vi "PusherClose.vi"   [LabVIEW 2014, in "PusherLib.lvlib"]
uses:
  PusherLib.lvlib
  PusherRefs.ctl
types:
  T1 = typedef "PusherLib.lvlib/PusherRefs.ctl" = enum16{"PusherLeft", "PusherRight", "PusherStringPot"}
  T2 = typedef "WPI_MotorControlDeviceRef.ctl" = cluster{"DeviceStatus":errorcluster, "Type":T3, "PWM":cluster{"Controller":T4, "PWM Channel":T5, "DeadBand":T6}, "CAN":cluster{"Device Number":u8, "Control Mode":T7, "Semaphore":T8, "Max Vout":dbl, "TalonSRX Control Mode":T9}, "Invert":bool, "TransformRef":T10, "InvTransformRef":T10}
  T3 = typedef "WPI_MotorControlType.ctl" = enum16{"PWM", "CAN", "CANTalonSRX"}
  T4 = typedef "FPGA_TypedefDigitalModule.ctl" = enum16{"Controller 1"}
  T5 = typedef "FPGA_DIOPWMChannel.ctl" = enum8{"PWM 0", "PWM 1", "PWM 2", "PWM 3", "PWM 4", "PWM 5", "PWM 6", "PWM 7", "PWM 8", "PWM 9", "PWM MXP 0", "PWM MXP 1", "PWM MXP 2", "PWM MXP 3", "PWM MXP 4", "PWM MXP 5", "PWM MXP 6", "PWM MXP 7", "PWM MXP 8", "PWM MXP 9", "Invalid"}
  T6 = typedef "WPI_PWMDeadband.ctl" = cluster{"Name":string, "maxPositivePwm":i32, "minPositivePwm":i32, "centerPwm":i32, "maxNegativePwm":i32, "minNegativePwm":i32, "angularRange":u16}
  T7 = typedef "WPI_CANJaguar_ControlMode.ctl" = enum8{"Percent VBus", "Current", "Speed", "Position", "Voltage"}
  T8 = typedef "Semaphore RefNum" = refnum<k1>
  T9 = typedef "WPI_CANTalonSRX_APIControlMode.ctl" = enum8{"Percent VBus", "Speed", "Position", "Slave", "Unchanged / Invalid"}
  T10 = typedef "WPI_PWMTransform_ConPane.ctl" = refnum<vi>
  T11 = typedef "WPI_PotentiometerDevRef.ctl" = cluster{"DevStatus":errorcluster, "Controller":T12, "Analog Channel":T13, "Invert Output":bool}
  T12 = typedef "FPGA_TypedefAnalogModule.ctl" = enum16{"Controller 1"}
  T13 = typedef "FPGA_AIChannel.ctl" = enum8{"AI 0", "AI 1", "AI 2", "AI 3", "AI MXP 0", "AI MXP 1", "AI MXP 2", "AI MXP 3", "Invalid"}
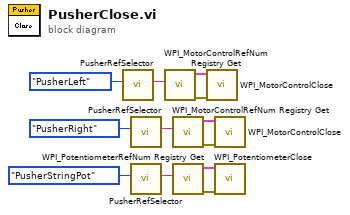
[diagram p0: block diagram]
diagram:
  n1 = call "PusherRefSelector.vi"("PusherRefs"=PusherRefs."PusherLeft") -> ("Refnum"=w9:string)  [unwired: 10 in]
  n2 = call "PusherRefSelector.vi"("PusherRefs"=PusherRefs."PusherRight") -> ("Refnum"=w8:string)  [unwired: 10 in]
  n3 = call "PusherRefSelector.vi"("PusherRefs"=PusherRefs."PusherStringPot") -> ("Refnum"=w1:string)  [unwired: 10 in]
  n4 = call <vilib>:"WPI_MotorControlRefNum Registry Get.vi"("refnum name"=w9) -> ("error out"=w11:errorcluster, "MotorControlDevRef"=w10:T2)  [unwired: 9 in]
  n5 = call <vilib>:"WPI_MotorControlRefNum Registry Get.vi"("refnum name"=w8) -> ("error out"=w6:errorcluster, "MotorControlDevRef"=w7:T2)  [unwired: 9 in]
  n6 = call <vilib>:"WPI_PotentiometerRefNum Registry Get.vi"("refnum name"=w1) -> ("error out"=w4:errorcluster, "PotDevRef"=w3:T11)  [unwired: 9 in]
  n7 = call <vilib>:"WPI_MotorControlClose.vi"("error in (no error)"=w11, "MotorControlDevRef"=w10) -> ()  [unwired: 9 in, 1 out]
  n8 = call <vilib>:"WPI_MotorControlClose.vi"("error in (no error)"=w6, "MotorControlDevRef"=w7) -> ()  [unwired: 9 in, 1 out]
  n9 = call <vilib>:"WPI_PotentiometerClose.vi"("error in"=w4, "PotDevRef"=w3) -> ()  [unwired: 9 in, 1 out]
